vi "Dashboard Main.vi"() -> ()   [LabVIEW 2014]
uses:
  <vilib>/event_ctls.llb/eventvkey.ctl
  <vilib>/Rock Robotics/WPI/Dashboard/WPI_DashboardLogging Global.vi
  <vilib>/Rock Robotics/Network Tables/SD Write Number.vi
  <vilib>/Rock Robotics/Network Tables/SD Write Boolean.vi
  <vilib>/Rock Robotics/Network Tables/SD Read String.vi
  <vilib>/Utility/config.llb/Write Key (String).vi
  <vilib>/Utility/config.llb/Write Key (I32).vi
  <vilib>/Utility/config.llb/NI_LVConfig.lvlib
panel:
  in  "TCP":refnum<k5>
  in  "Rec Mode":enum32{"Stop", "Record", "Playback"}(radio)
  in  "Vision":u16(ring) items=["Camera Off", "USB Camera SW", "USB Camera HW", "IP Camera"]
  out "Camera IP":string
  out "Image Message":string="Timeout in Camera Communications"
  in  "Dashboard Tab":T1(tab)
  in  "CPS":dbl
  in  "Precision":bool
  out "?":string
  out "?":string
  out "?":string
  out "?":string
  out "?":string
  out "?":string
  in  "?":bool
  in  "?":bool
  in  "?":bool
  in  "Precision":dbl(slide) scale=0.0..100.0
  in  "Camera Settings":T2={"Frame Rate"=30, "Compression"=30, "Size"=1} {"Frame Rate" scale=1.0..30.0; "Size" items=["640x480", "320x240", "160x120"]}
  out "MotorChart R":cluster{"Numeric":dbl, "Numeric":dbl}(graph)
  out "MotorChart L":T3(graph)
  out "MotorSliders R":cluster{"MotorSlide1":dbl, "MotorSlide2":dbl} {"MotorSlide2" scale=-1.0..1.0 scale format="%#_2e"; "MotorSlide1" scale=-1.0..1.0 scale format="%#_2e"}
  out "MotorSliders L":T4 {"MotorSlide4 2" scale=0.0..14.0 scale format="%#_2e"; "MotorSlide2" scale=-1.0..1.0 scale format="%#_2e"; "MotorSlide1" scale=-1.0..1.0 scale format="%#_2e"}
  out "?":dbl(knob) scale=0.0..360.0
  out "JS1 Z":dbl(slide) scale=-1.0..1.0 scale format="%#_2e"
  out "JS1 Graph":cluster{"X":dbl, "Y":dbl}[](graph)
  out "JS1 Buttons":T5
  out "JS2 Z":dbl(slide) scale=-1.0..1.0 scale format="%#_2e"
  out "JS2 Graph":cluster{"X":dbl, "Y":dbl}[](graph)
  out "JS2 Buttons":T5
  out "Mode":T6(ring)=enum."Auto Disabled"
  in  "DB Camera Config":bool
  out "fps":dbl format="%#.1g"
  out "Mbps":dbl format="%#.1g"
  out "Mbps 2":bool
  in  "DB/String 9":string
  in  "DB/String 8":string
  in  "DB/String 7":string
  in  "DB/String 6":string
  in  "DB/String 5":string
  in  "DB/String 4":string
  in  "DB/String 3":string
  in  "DB/String 2":string
  in  "DB/String 1":string
  in  "DB/String 0":string
  in  "DB/Slider 0":dbl(slide) scale=0.0..5.0
  in  "DB/Slider 1":dbl(slide) scale=0.0..5.0
  in  "DB/Slider 2":dbl(slide) scale=0.0..5.0
  in  "DB/Slider 3":dbl(slide) scale=0.0..5.0
  out "DB/LED 3":bool
  out "DB/LED 2":bool
  out "DB/LED 1":bool
  out "DB/LED 0":bool
  in  "DB/Button 3":bool
  in  "DB/Button 2":bool
  in  "DB/Button 1":bool
  in  "DB/Button 0":bool caption="New Name"
  in  "Test Slider":dbl(slide) scale=0.0..100.0 scale format="%#_3g"
  in  "On/Off":bool caption="Solenoid"
  in  "Test Name":u16(ring) items=["Select the test to run...", "Example Test", "-------------------------------", "List of tests is built in robot code.", "Replace with your own automated tests."]
  in  "Test Tree":string(tree)
  in  "Motor":cluster{"Value":dbl, "Enable":bool} {"Value" scale=-1.0..1.0 scale format="%#_3g"}
  out "Progress":T7 {"Test Progress" scale=0.0..100.0}
  in  "Rev/Fwd":cluster{"Forward":bool, "Reverse":bool}
  in  "Test Ring":u16(ring) items=["Monochrome", "Color"]
  in  "Listbox":i32(listbox)
  out "Tree":string(tree)
  in  "Invert Z":bool
  in  "Invert Y":bool
  in  "Invert X":bool
  out "Camera Image":T8(plugin-control)
  out "Boolean":bool
  # "Left"
  # "Front"
  # "Right"
  # "Battery"
  # "This tab is a great place for autonomous settings and robot-specific values.\nPlace controls and indicators inside this tab and match name to\nDashboard Variables on robot. You can also delete this comment."
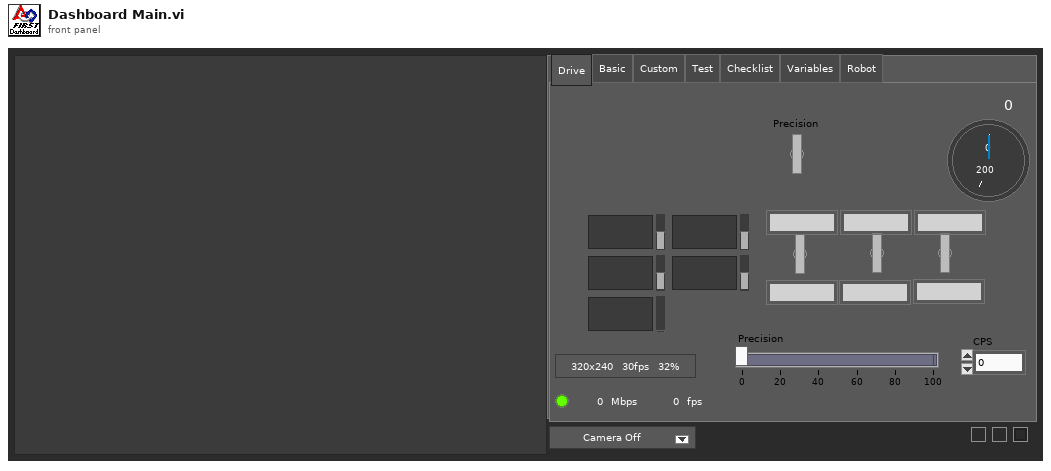
[diagram p1: front panel]
types:
  T1 = enum32{"Drive", "Basic", "Custom", "Test", "Checklist", "Variables", "Robot"}
  T2 = cluster{"Frame Rate":i32, "Compression":i32, "Size":u16}
  T3 = cluster{"Numeric":dbl, "Numeric":dbl, "Battery V":dbl}
  T4 = cluster{"MotorSlide1":dbl, "MotorSlide2":dbl, "MotorSlide4 2":dbl}
  T5 = cluster{bool, bool, bool, bool, bool, bool, bool, bool, bool, bool, bool, bool}
  T6 = enum8{"Tele-Op Disabled", "Tele-Op Enabled", "Auto Disabled", "Auto Enabled", "Test Disabled", "Test Enabled", "Disconnected", "No Code", "E-Stop"}
  T7 = cluster{"Test Progress":u8, "Test Progress Text":string}
  T8 = typedef "IMAQ Image.ctl" = refnum<image>
  T9 = enum32{"Drive", "Basic", "Custom", "Test", "Checklist", "Variables"}
  T10 = typedef "Image Type" = u32
  T11 = cluster{"Camera Image":refnum<vi>, "Dashboard Tab":refnum<vi>, "Boolean":refnum<vi>, "Vision":refnum<vi>, "Rec Mode":refnum<vi>, "Test Slider":refnum<vi>, "On/Off ":refnum<vi>, "Test Ring":refnum<vi>, "Rev/Fwd":refnum<vi>, "Test Name":refnum<vi>, "Motor":refnum<vi>, "Progress":refnum<vi>, "CheckList":refnum<vi>, "Tree":refnum<vi>, "Test Tree":refnum<vi>}
  T12 = typedef "NI_LVConfig.lvlib/Config Data RefNum.ctl" = refnum<k1>
  T13 = cluster{"Error Strings":string, "Disable Counts":cluster{u16, u16}, "Rail Faults":cluster{u16, u16, u16}, "Robot IP":string, "DB Mode":u8, "Event Info":cluster{"Name":string, "Type":u8, "Number":u16, "Replay":u8}, "Camera Addr":string}
  T14 = cluster{"Storage":cluster{"Disk Free":u64, "RAM Block":u32, "RAM free":u32}, "CPU Utilization":cluster{"CPU % ISR":sgl, "CPU % Time Crit":sgl, "CPU % Timed Str":sgl, "CPU % High":sgl, "CPU % Above":sgl, "CPU % Normal":sgl, "CPU % Low":sgl}, "CAN":cluster{"% Bus Utilization":sgl, "Bus Off Cnt":u32, "TX_FIFO Full Cnt":u32, "Receive Error Cnt":u8, "Transmit Error Cnt":u8}, "HID":cluster{"HID Outputs":u32, "Rumble Low":u16, "Rumble High":u16}[]}
  T15 = cluster{"Status bits":cluster{"Test Mode":bool, "Autonomous":bool, "Enabled":bool, "Code Start":bool, "Brownout":bool, "Reserved 2":bool, "Reserved 3":bool, "E-Stop":bool}, "Code Trace":cluster{"Disabled":bool, "TeleOp":bool, "Auto":bool, "Test":bool}, "Controller Type":enum16{"unknown", "cRIO", "roboRio"}, "Code?":enum16{"unknown", "noCode", "code"}, "Battery V":dbl}
  T16 = cluster{"Control Bits":cluster{"TestMode":bool, "Autonomous":bool, "Enabled":bool, "FMS Present":bool, bool, bool, bool, "E-Stop":bool}, "Team Station ":u8, "Countdown":sgl, "Joystick Values":cluster{"Axes":dbl[], "Buttons":bool[], "POVs":i16[]}[]}
  T17 = cluster{"Axes":dbl[], "Buttons":bool[], "POVs":i16[]}[]
  T18 = cluster{"Axes":dbl[], "Buttons":bool[], "POVs":i16[]}
  T19 = cluster{"Buttons[0]":bool, "Buttons[1]":bool, "Buttons[2]":bool, "Buttons[3]":bool, "Buttons[4]":bool, "Buttons[5]":bool, "Buttons[6]":bool, "Buttons[7]":bool, "Buttons[8]":bool, "Buttons[9]":bool, "Buttons[10]":bool, "Buttons[11]":bool}
  T20 = cluster{"Operation":enum16{"Update", "Clear"}, "Color Box":u32}[]
  T21 = typedef "eventvkey.ctl" = enum16{"ASCII", "Enter", "Return", "Shift", "Ctrl", "Alt", "Cmd", "Opt", "Caps", "NumLock", "Clear", "Break", "Up", "Down", "Left", "Right", "Insert", "Delete", "Home", "End", "PageUp", "PageDown", "Escape", "Help", "Pause", "ScrollLock", "F1", "F2", "F3", "F4", "F5", "F6", "F7", "F8", "F9", "F10", "F11", "F12", "F13", "F14", "F15", "F16", "F17", "F18", "F19", "F20", "F21", "F22", "F23", "F24", "Play", "VolumeUp", "VolumeDown", "Mute", "Two Byte Char"}
  T22 = cluster{"Image Size":bool, "Image Type":bool, "Pixel Value":bool, "ROI Information":bool, "Zoom Factor":bool}
  T23 = enum8{"Enabled", "Disabled", "Disabled and Grayed Out"}
  T24 = cluster{"Operation":enum16{"Update", "Clear"}, "Color Box":u32}
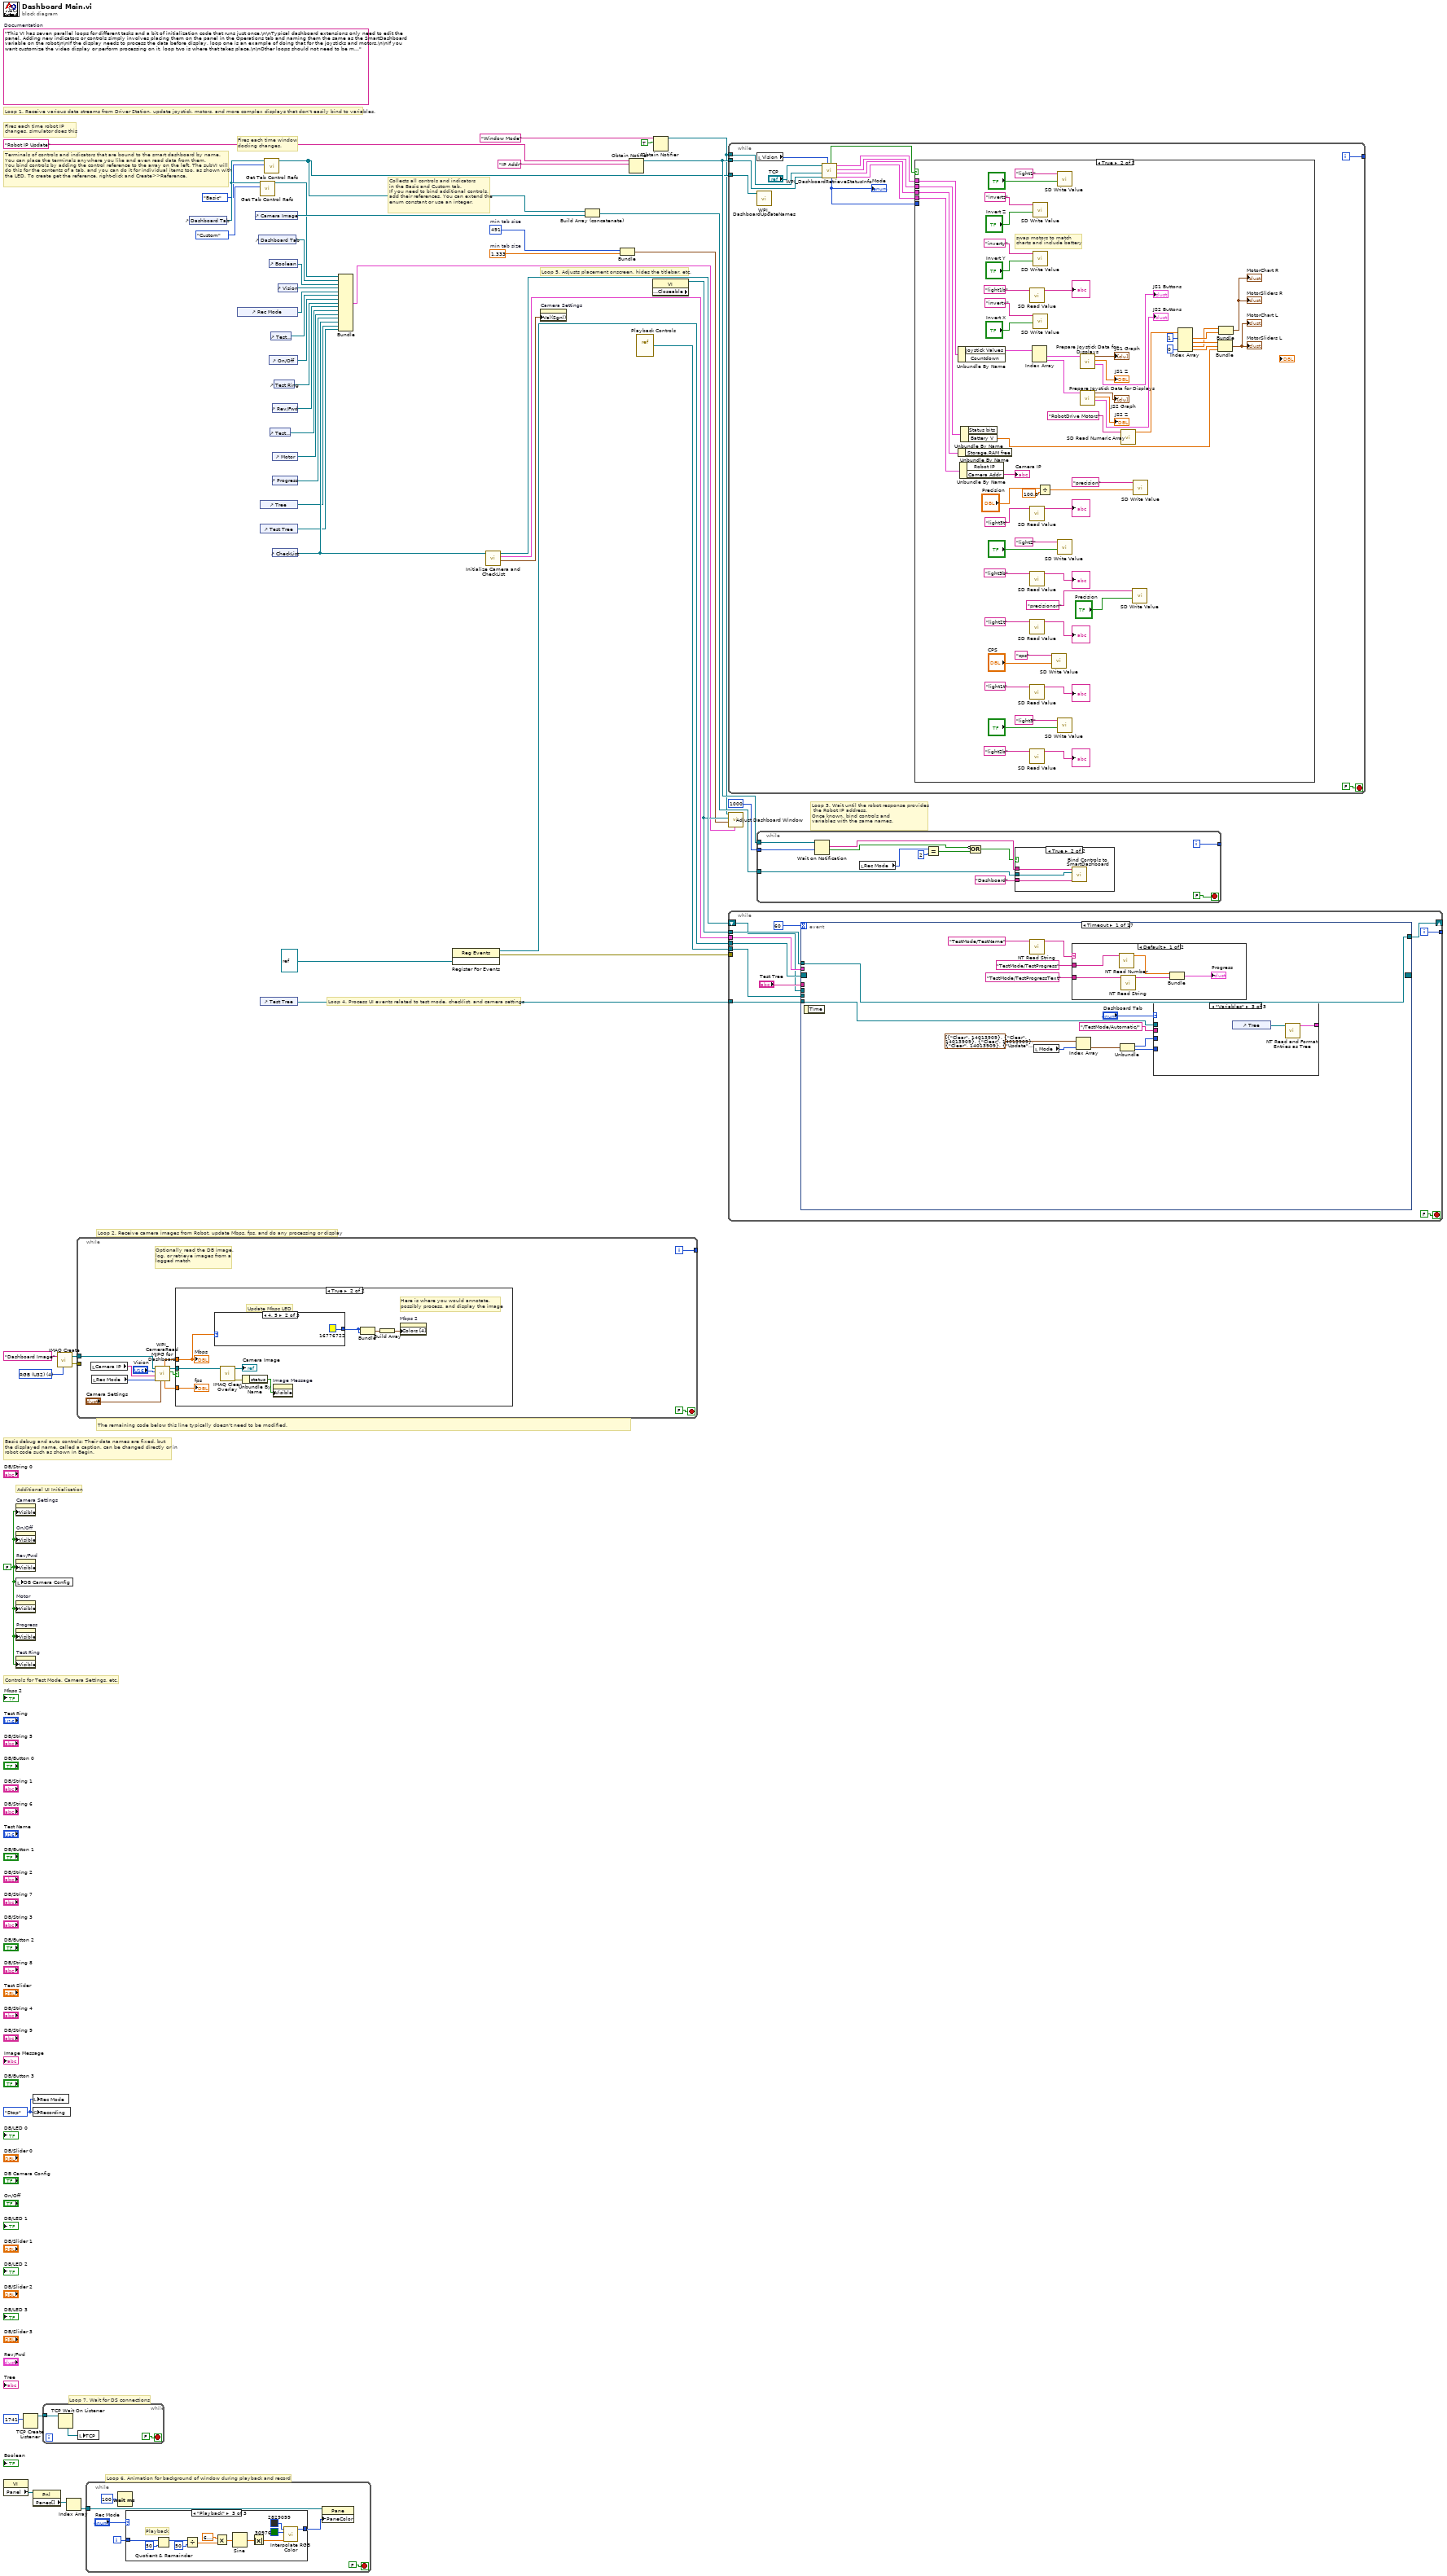
[diagram p0: block diagram]
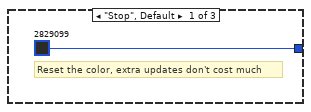
[diagram p3: hidden frame]
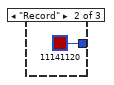
[diagram p4: hidden frame]
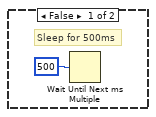
[diagram p6: hidden frame]
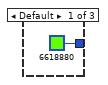
[diagram p7: hidden frame]
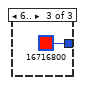
[diagram p8: hidden frame]
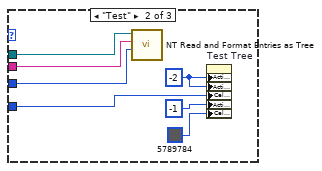
[diagram p10: hidden frame]
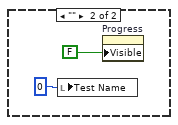
[diagram p11: hidden frame]
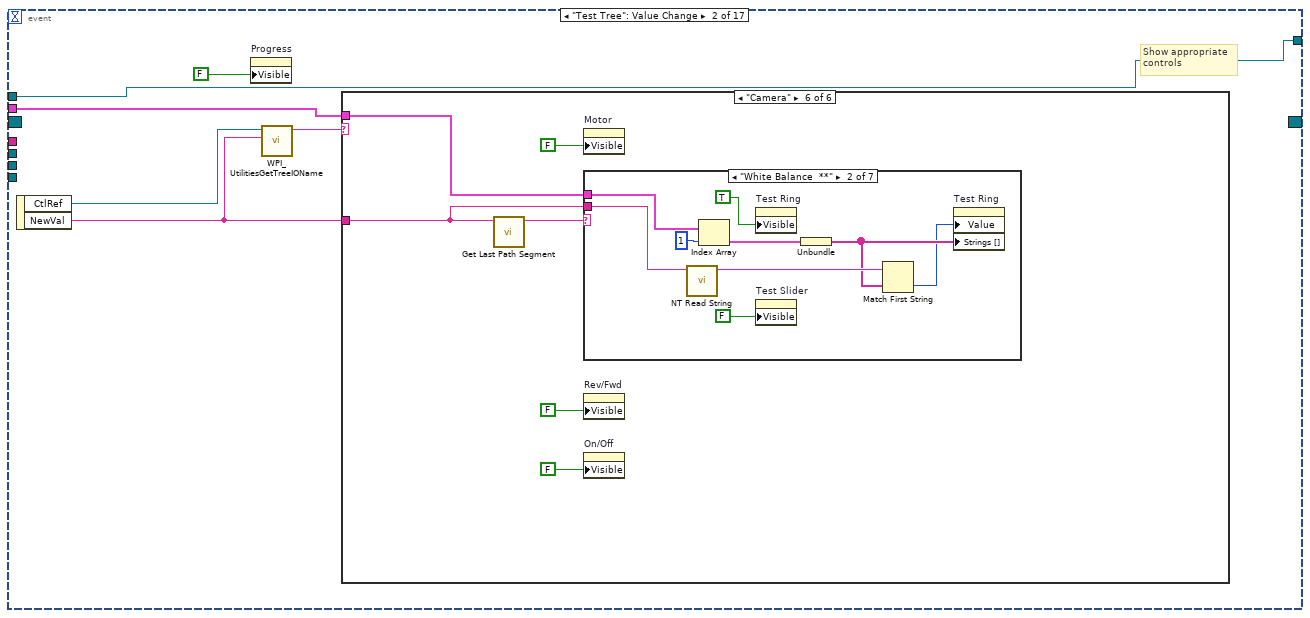
[diagram p12: hidden frame]
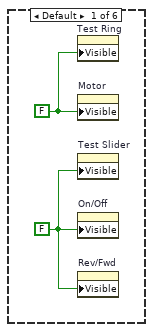
[diagram p13: hidden frame]
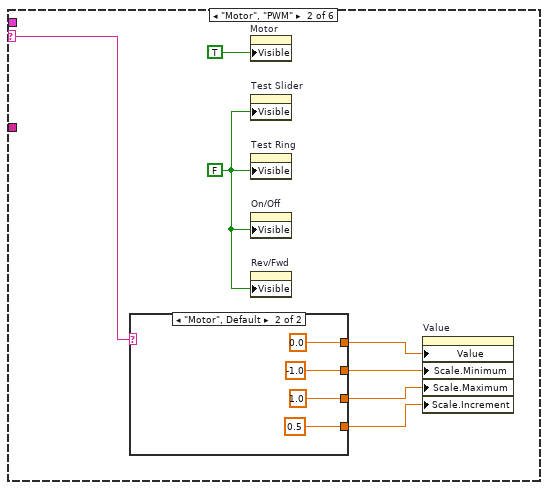
[diagram p14: hidden frame]
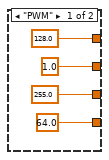
[diagram p15: hidden frame]
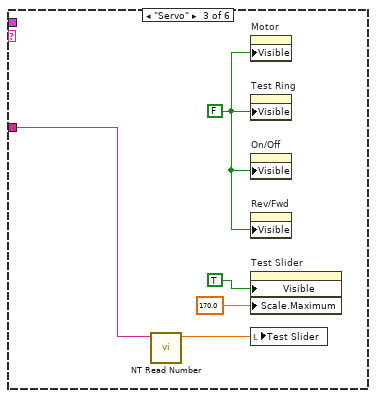
[diagram p16: hidden frame]
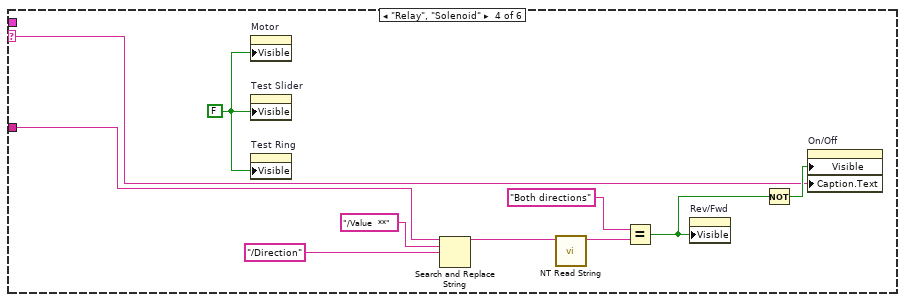
[diagram p17: hidden frame]
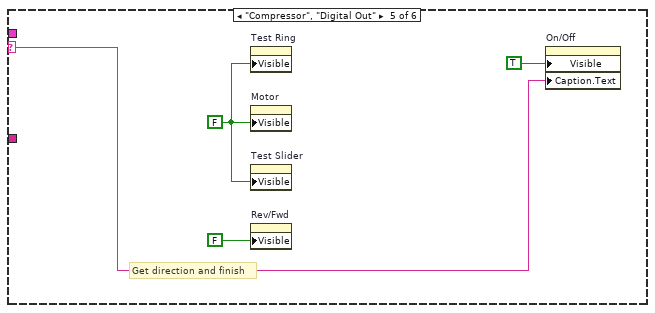
[diagram p18: hidden frame]
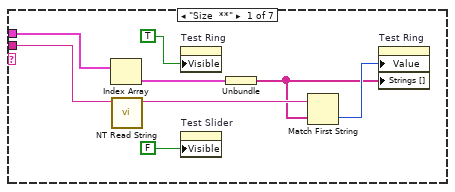
[diagram p19: hidden frame]
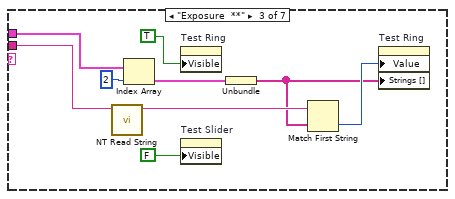
[diagram p20: hidden frame]
diagram:
  w24 = 491  # min tab size
  w23 = 1.333  # min tab size
  w32 = enum32{"Stop", "Record", "Playback"}."Stop" ("Rec Mode")
  w6 = FALSE ("Visible")
  (unwired) "This VI has seven parallel loops for different tasks and a bit of initialization code that runs just once.\n\nTypical dashboard extensions only need to edit the panel. Adding new indicators or controls simply involves placing them on the panel in the Operations tab and naming them the same as the SmartDashboard variable on the robot\n\nIf the display needs to process the data before display, loop one is an example of doing that for the joysticks and motors.\n\nIf you want customize the video display or perform processing on it, loop two is where that takes place.\n\nOther loops should not need to be modified. They are pretty standard, and document the task they perform."  # Documentation
  w52 = T10 4 items=["Grayscale (U8)", "Grayscale (I16)", "Grayscale (SGL)", "Complex (CSG)", "RGB (U32)", "HSL (U32)", "RGB (U64)"] ("Image Type")
  # "Loop 7. Wait for DS connections"
  # "Basic debug and auto controls: Their data names are fixed, but\nthe displayed name, called a caption, can be changed directly or in\nrobot code such as shown in Begin."
  # "Controls for Test Mode, Camera Settings, etc."
  # "Additional UI Initialization"
  # "Loop 6. Animation for background of window during playback and record"
  # "Fires each time robot IP\nchanges, simulator does this"
  # "Fires each time window\ndocking changes."
  # "Collects all controls and indicators\nin the Basic and Custom tab.\nIf you need to bind additional controls,\nadd their references. You can extend the\nenum constant or use an integer."
  # "The remaining code below this line typically doesn't need to be modified."
  # "Loop 4. Process UI events related to test mode, checklist, and camera settings"
  # "Terminals of controls and indicators that are bound to the smart dashboard by name.\nYou can place the terminals anywhere you like and even read data from them.\nYou bind controls by adding the control reference to the array on the left. The subVI will\ndo this for the contents of a tab, and you can do it for individual items too, as shown with\nthe LED. To create get the reference, right-click and Create>>Reference."
  # "Loop 3. Wait until the robot response provides\n the Robot IP address.\nOnce known, bind controls and\nvariables with the same names."
  # "Loop 5. Adjusts placement onscreen, hides the titlebar, etc."
  # "Loop 1. Receive various data streams from Driver Station, update joystick, motors, and more complex displays that don't easily bind to variables."
  # "Loop 2. Receive camera images from Robot, update Mbps, fps, and do any processing or display"
  n1 = property class="VI"() -> ("Panel"=w39:refnum<vi>)  [unwired: 2 in, 2 out]
  n2 = property on="Camera Settings" class="Clust (strict)"("Visible"=w6) -> ()  [unwired: 2 in, 2 out]
  n3 = property on="On/Off" class="Bool (strict)"("Visible"=w6) -> ()  [unwired: 2 in, 2 out]
  n4 = property on="Rev/Fwd" class="Clust (strict)"("Visible"=w6) -> ()  [unwired: 2 in, 2 out]
  n5 = local write "DB Camera Config"(w6) -> ()
  n6 = property on="Motor" class="Clust (strict)"("Visible"=w6) -> ()  [unwired: 2 in, 2 out]
  n7 = property on="Progress" class="Clust (strict)"("Visible"=w6) -> ()  [unwired: 2 in, 2 out]
  n8 = property on="Test Ring" class="Ring (strict)"("Visible"=w6) -> ()  [unwired: 2 in, 2 out]
  n9 = TCP Create Listener(10:u16 1741 ("timeout ms (25000)")) -> (3:w1:refnum<k5>)  [unwired: 4 in, 2 out]
  n10 = local write "Rec Mode"(w32) -> ()
  n11 = global write "WPI_DashboardLogging Global.vi" "Recording"(w32) -> ()
  n12 = property class="Pnl"(reference=w39) -> ("Panes[]"=w40:refnum<vi>[])  [unwired: 1 in, 2 out]
  n13 = while {
    tunnel: w1 -> [w54]
    stop <- FALSE stop-if-true
    n14 = TCP Wait On Listener(11:w54) -> (4:w53:refnum<k5>)  [unwired: 3 in, 4 out]
    n15 = local write "TCP"(w53) -> ()
  }
  n16 = call "IMAQ Create"("Image Name"="Dashboard Image", "Image Type"=w52) -> ("New Image"=w50:T8, "error out"=w49:errorcluster)  [unwired: 2 in, 1 out]
  n17 = Index Array(array=w40) -> (element=w38:refnum<vi>)  [unwired: 1 in]
  n18 = while {
    tunnel: w50 -> [w64]
    tunnel: w49 -> [_]
    tunnel: [w65] -> _
    i -> [w65]
    stop <- FALSE stop-if-true
    # "Optionally read the DB image,\nlog, or retrieve images from a\nlogged match"
    n19 = local read "Camera IP"() -> (w56:string)
    n20 = local read "Rec Mode"() -> (w58:enum32{"Stop", "Record", "Playback"})
    n21 = call <vilib>:"WPI_CameraRead MJPG for Dashboard.vi"("Camera Settings"="Camera Settings", "Rec Mode"=w58, "Camera IP"=w56, "Camera Mode"="Vision", "Refnum in"=w64) -> ("Active"=w62:bool, "Refnum out"=w63:T8, "FPS"=w61:dbl, "Bandwidth (Mbps)"=w60:dbl)  [unwired: 3 in]
    n22 = case shown="True" w62 {
      tunnel: w63 -> [_ w71]
      tunnel: w60 -> [_ w70]
      tunnel: w61 -> [_ w68]
      frame False {
        # "Sleep for 500ms"
        n23 = Wait Until Next ms Multiple(millisecond multiple=u32 500) -> ()  [unwired: 1 out]
      }
      frame True {
        # "Here is where you would annotate,\npossibly process, and display the image"
        # "Update Mbps LED"
        n24 = case shown="4, 5" w70 {
          tunnel: [u32 6618880 ("Color Box") u32 16776722 ("Color Box") u32 16716800 ("Color Box")] -> w72
          frame Default {
          }
          frame 4, 5 {
          }
          frame 6.. {
          }
        }
        n25 = call "IMAQ Clear Overlay"("Image"=w71) -> ("error out"=w75:errorcluster, "Image Out"=→"Camera Image":T8)  [unwired: 2 in, 7 out]
        n26 = Unbundle By Name(w75) -> ("status"=w76:bool)
        n27 = property on="Image Message" class="Str"("Visible"=w76) -> ()  [unwired: 2 in, 2 out]
        n28 = Bundle("Color Box"=w72, "Color Box"=w72) -> (w74:cluster{"Color Box":u32, "Color Box":u32})  [unwired: 1 out]
        n29 = Build Array(w74) -> (w73:cluster{"Color Box":u32, "Color Box":u32}[])
        n30 = property on="Mbps 2" class="Bool (strict)"("Colors [4]"=w73) -> ()  [unwired: 2 in, 2 out]
        "Mbps" <- w70
        "fps" <- w68
      }
    }
  }
  n31 = while {
    tunnel: w38 -> [w81]
    i -> [w84]
    stop <- FALSE stop-if-true
    n32 = Wait (ms)(milliseconds to wait=u32 100) -> ()  [unwired: 1 out]
    n33 = case shown="\"Playback\"" "Rec Mode" {
      tunnel: w84 -> [_ _ w99]
      tunnel: [u32 2829099 ("Base Color") u32 11141120 ("Target Color") w88] -> w80
      frame "Stop", Default {
        # "Reset the color, extra updates don't cost much"
      }
      frame "Record" {
      }
      frame "Playback" {
        # "Playback"
        n34 = Quotient & Remainder(x=w99, y=u32 50 ("milliseconds to wait")) -> (x-y*floor(x/y)=w95:u32)  [unwired: 1 out]
        n35 = Divide(x=w95, y=u32 50 ("milliseconds to wait")) -> (x/y=w92:dbl)
        n36 = Multiply(x=6.283185307179586, y=w92) -> (x*y=w97:dbl)
        n37 = Sine(x=w97) -> (sin(x)=w96:dbl)
        n38 = Absolute Value(x=w96) -> (abs(x)=w89:dbl)
        n39 = call "Interpolate RGB Color.vi"("Proportion"=w89, "Target Color"=u32 30976, "Base Color"=u32 2829099) -> ("Result Color"=w88:u32)  [unwired: 8 in]
      }
    }
    n40 = property class="Pane"(reference=w81, "PaneColor"=w80) -> ()  [unwired: 1 in, 2 out]
  }
  n41 = control-ref of="Dashboard Tab"() -> (w30:refnum<vi>)
  n42 = control-ref of="Rec Mode"() -> (w12:refnum<vi>)
  n43 = control-ref of="Camera Image"() -> (w27:refnum<vi>)
  n44 = control-ref of="Dashboard Tab"() -> (w26:refnum<vi>)
  n45 = control-ref of="Tree"() -> (w16:refnum<vi>)
  n46 = control-ref of="Test Tree"() -> (w15:refnum<vi>)
  n47 = control-ref of="Test Tree"() -> (w41:refnum<vi>)
  n48 = call <vilib>:"Get Tab Control Refs.vi"("Page Index"=T9."Custom" ("Dashboard Tab"), "TabControl in"=w30) -> ("ControlsOnPage"=w29:refnum<vi>[])  [unwired: 9 in]
  n49 = call <vilib>:"Get Tab Control Refs.vi"("Page Index"=T9."Basic" ("Dashboard Tab"), "TabControl in"=w30) -> ("ControlsOnPage"=w4:refnum<vi>[])  [unwired: 9 in]
  n50 = control-ref of="Boolean"() -> (w21:refnum<vi>)
  n51 = control-ref of="On/Off"() -> (w10:refnum<vi>)
  n52 = control-ref of="Test Name"() -> (w14:refnum<vi>)
  n53 = control-ref of="Test Slider"() -> (w11:refnum<vi>)
  n54 = control-ref of="Rev/Fwd"() -> (w8:refnum<vi>)
  n55 = control-ref of="Motor"() -> (w13:refnum<vi>)
  n56 = control-ref of="Progress"() -> (w7:refnum<vi>)
  n57 = control-ref of="CheckList"() -> (w17:refnum<vi>)
  n58 = control-ref of="Test Ring"() -> (w9:refnum<vi>)
  n59 = control-ref of="Vision"() -> (w25:refnum<vi>)
  n60 = Bundle("Camera Image"=w27, "Dashboard Tab"=w26, "Boolean"=w21, "Vision"=w25, "Rec Mode"=w12, "Test Slider"=w11, "On/Off"=w10, "Test Ring"=w9, "Rev/Fwd"=w8, "Test Name"=w14, "Motor"=w13, "Progress"=w7, "CheckList"=w17, "Tree"=w16, "Test Tree"=w15) -> (w18:T11)  [unwired: 1 in]
  n61 = register-events(refnum<vi> refnum) -> (reference out=w36:refnum<event-registration>, error out=w35:errorcluster)  [unwired: 2 in]
  n62 = call "Initialize Camera and CheckList.vi"("ListBox in"=w17) -> ("Cluster"=w43:cluster{"value":i32, "value":i32, "index":i32}, "Array"=w44:cluster{string[]}[], "File Refnum"=w42:T12)  [unwired: 8 in]
  n63 = property on="Camera Settings" class="Clust (strict)"("Val(Sgnl)"=w43) -> ()  [unwired: 2 in, 2 out]
  n64 = Build Array (concatenate)(w4, w29) -> (w28:refnum<vi>[])
  n65 = Bundle("min tab size"=w24, "min tab size"=w23) -> (w22:cluster{"min tab size":i32, "min tab size":dbl})  [unwired: 1 in]
  n66 = Obtain Notifier(name (unnamed)="Robot IP Update", notification data type="IP Addr" ("name (unnamed)")) -> (notifier out=w5:refnum<notifier>)  [unwired: 2 in, 2 out]
  n67 = vi-ref "Playback Controls.vi"() -> (w37:refnum<vi>)
  n68 = property class="VI" props=["Front Panel.Closeable"]() -> (reference out=w31:refnum<vi>)  [unwired: 2 in, 2 out]
  n69 = Obtain Notifier(name (unnamed)="Window Mode", notification data type=TRUE) -> (notifier out=w3:refnum<notifier>)  [unwired: 2 in, 2 out]
  n70 = while {
    tunnel: [w111] -> _
    tunnel: w5 -> [w105]
    tunnel: w4 -> [w104]
    tunnel: w3 -> [w100]
    i -> [w111]
    stop <- FALSE stop-if-true
    n71 = local read "Vision"() -> (w102:u16)
    n72 = call <vilib>:"WPI_DashboardUpdateNames.vi"("Controls on Tab"=w104) -> ()  [unwired: 11 in]
    n73 = call <vilib>:"WPI_DashboardRetrieveStatusInfo.vi"("Vision"=w102, "Binding Refnum"=w105, "Window Mode Notifier"=w100, "TCP Cnx"="TCP") -> ("Power and Errors"=w106:T13, "Robot Metrics"=w109:T14, "Status Info"=w110:T15, "Control Info"=w107:T16, "Robot Mode"=w103:T6, "Process?"=w108:bool)  [unwired: 2 in]
    "Mode" <- w103
    n74 = case shown="True" w108 {
      tunnel: w110 -> [_ w169]
      tunnel: w109 -> [_ w168]
      tunnel: w107 -> [_ w167]
      tunnel: w106 -> [_ w166]
      tunnel: w103 -> [_ _]
      frame False {
      }
      frame True {
        # "swap motors to match\ncharts and include battery"
        n75 = Unbundle By Name(w167) -> ("Joystick Values"=w154:T17)  [unwired: 1 out]
        n76 = Unbundle By Name(w168) -> ()  [unwired: 1 out]
        n77 = Unbundle By Name(w166) -> ("Camera Addr"=→"Camera IP":string)  [unwired: 1 out]
        n78 = Unbundle By Name(w169) -> ("Battery V"=w155:dbl)  [unwired: 1 out]
        n79 = call-poly <vilib>:"SD Read Value.vi"("Name"="light1b") -> ("String"=→"?":string)  [unwired: 8 in, 2 out]
        n80 = call-poly <vilib>:"SD Read Value.vi"("Name"="light3t") -> ("String"=→"?":string)  [unwired: 8 in, 2 out]
        n81 = call-poly <vilib>:"SD Read Value.vi"("Name"="light3b") -> ("String"=→"?":string)  [unwired: 8 in, 2 out]
        n82 = call-poly <vilib>:"SD Read Value.vi"("Name"="light2t") -> ("String"=→"?":string)  [unwired: 8 in, 2 out]
        n83 = call-poly <vilib>:"SD Read Value.vi"("Name"="light1t") -> ("String"=→"?":string)  [unwired: 8 in, 2 out]
        n84 = call-poly <vilib>:"SD Read Value.vi"("Name"="light2b") -> ("String"=→"?":string)  [unwired: 8 in, 2 out]
        n85 = Index Array(array=w154) -> (element #1=w153:T18, element #2=w148:T18)  [unwired: 2 in]
        n86 = call-poly <vilib>:"SD Write Value.vi"("Boolean"="Invert Z", "Name"="invertz") -> ()  [unwired: 8 in, 2 out]
        n87 = call-poly <vilib>:"SD Write Value.vi"("Boolean"="Invert Y", "Name"="inverty") -> ()  [unwired: 8 in, 2 out]
        n88 = call-poly <vilib>:"SD Write Value.vi"("Boolean"="Invert X", "Name"="invertx") -> ()  [unwired: 8 in, 2 out]
        n89 = Divide(x="Precision", y=100.0) -> (x/y=w143:dbl)
        n90 = call-poly <vilib>:"SD Write Value.vi"("Numeric"="CPS", "Name"="cps") -> ()  [unwired: 8 in, 2 out]
        n91 = call-poly <vilib>:"SD Write Value.vi"("Boolean"="?", "Name"="light1") -> ()  [unwired: 8 in, 2 out]
        n92 = call-poly <vilib>:"SD Write Value.vi"("Boolean"="?", "Name"="light2") -> ()  [unwired: 8 in, 2 out]
        n93 = call-poly <vilib>:"SD Write Value.vi"("Boolean"="?", "Name"="light3") -> ()  [unwired: 8 in, 2 out]
        n94 = call "Prepare Joystick Data for Displays.vi"("Joystick Values"=w153) -> ("Buttons"=→"JS1 Buttons":T19, "Z Axis"=→"JS1 Z":dbl, "Cartesian Data"=→"JS1 Graph":cluster{"X axis":dbl, "X axis":dbl}[])  [unwired: 8 in]
        n95 = call "Prepare Joystick Data for Displays.vi"("Joystick Values"=w148) -> ("Buttons"=→"JS2 Buttons":T19, "Z Axis"=→"JS2 Z":dbl, "Cartesian Data"=→"JS2 Graph":cluster{"X axis":dbl, "X axis":dbl}[])  [unwired: 8 in]
        n96 = call <vilib>:"SD Read Numeric Array.vi"("Name"="RobotDrive Motors") -> ("Numeric Array"=w157:dbl[])  [unwired: 8 in, 2 out]
        n97 = call-poly <vilib>:"SD Write Value.vi"("Boolean"="Precision", "Name"="precisionon") -> ()  [unwired: 8 in, 2 out]
        n98 = call-poly <vilib>:"SD Write Value.vi"("Numeric"=w143, "Name"="precision") -> ()  [unwired: 8 in, 2 out]
        n99 = Index Array(array=w157, index #1=1, index #4=0) -> (element #1=w161:dbl, element #2=w162:dbl, element #3=w160:dbl, element #4=w165:dbl)  [unwired: 2 in]
        n100 = Bundle("Numeric"=w162, "Numeric"=w165, "Battery V"=w155) -> (→"MotorChart L" →"MotorSliders L":T3)  [unwired: 1 in]
        n101 = Bundle("Numeric"=w160, "Numeric"=w161) -> (→"MotorChart R" →"MotorSliders R":cluster{"Numeric":dbl, "Numeric":dbl})  [unwired: 1 in]
      }
    }
  }
  n102 = call "Adjust Dashboard Window.vi"("Sizing Refnums"=w18, "Size Constraints"=w22, "VI"=w31, "Notifier in"=w3) -> ()  [unwired: 8 in]
  n103 = while {
    tunnel: w44 -> [w177]
    shift-right: [w176] -> _
    shift-left: w42 -> [w175]
    tunnel: [w174] -> _
    tunnel: w41 -> [w173]
    tunnel: w37 -> [w172]
    tunnel: w36 -> [w171]
    tunnel: w35 -> [_]
    tunnel: w31 -> [w170]
    i -> [w174]
    stop <- FALSE stop-if-true
    n104 = event shown="[0] Timeout" {
      selector: w171 -> [_ _ _ _ _ _ _ _ _ _ _ _ _ _ _ _ _]
      dyn-events: [_ _ _ _ _ _ _ _ _ _ _ _ _ w415 _ _ _] -> _
      timeout: u32 60 ("milliseconds to wait") -> [_ _ _ _ _ _ _ _ _ _ _ _ _ _ _ _ _]
      tunnel: w173 -> [w189 _ _ _ _ _ _ _ _ _ _ _ _ _ _ _ _]
      tunnel: "Test Tree" -> [_ _ _ _ _ _ _ _ w384 w392 w394 w398 w406 _ _ _ _]
      tunnel: w177 -> [_ w211 _ _ _ _ w348 w378 _ _ _ _ _ _ _ _ _]
      tunnel: [w185 w210 w309 w314 w322 w334 w347 w371 w383 w390 w393 w397 w405 w417 w431 w432 w442] -> w176
      tunnel: w175 -> [w185 w210 w309 w314 w322 w334 w346 w371 w383 w390 w393 w397 w405 w417 w431 w432 w442]
      tunnel: w172 -> [_ _ _ _ _ _ _ _ _ _ _ _ _ w418 _ w435 _]
      tunnel: w170 -> [_ _ _ _ _ _ _ _ _ _ _ _ _ w413 _ _ _]
      event Timeout {
        n105 = event-data() -> ()  [unwired: 1 in, 1 out]
        n106 = call <vilib>:"NT Read String.vi"("Name"="TestMode/TestName") -> ("String"=w192:string)  [unwired: 9 in, 1 out]
        n107 = local read "Mode"() -> (w188:T6)
        n108 = case shown="Default" w192 {
          tunnel: "TestMode/TestProgress" ("Name") -> [w204 _]
          tunnel: "TestMode/TestProgressText" ("Name") -> [w203 _]
          frame Default {
            n109 = call <vilib>:"NT Read Number.vi"("Name"=w204) -> ("Numeric"=w205:dbl)  [unwired: 9 in, 1 out]
            n110 = call <vilib>:"NT Read String.vi"("Name"=w203) -> ("String"=w206:string)  [unwired: 9 in, 1 out]
            n111 = Bundle("Numeric"=w205, "String"=w206) -> (→"Progress":cluster{"Numeric":dbl, "String":string})  [unwired: 1 in]
          }
          frame "" {
            n112 = local write "Test Name"(u16 0) -> ()
            n113 = property on="Progress" class="Clust (strict)"("Visible"=FALSE) -> ()  [unwired: 2 in, 2 out]
          }
        }
        n114 = Index Array(array=T20 [{"Operation"=enum."Clear", "Color Box"=14013909}, {"Operation"=enum."Clear", "Color Box"=14013909}, {"Operation"=enum."Clear", "Color Box"=14013909}, {"Operation"=enum."Clear", "Color Box"=14013909}, {"Operation"=enum."Update", "Color Box"=14013909}, {"Operation"=enum."Update", "Color Box"=16777215}, {"Operation"=enum."Clear", "Color Box"=14013909}, {"Operation"=enum."Clear", "Color Box"=14013909}, {"Operation"=enum."Clear", "Color Box"=14013909}], index=w188) -> (element=w183:T24)
        n115 = Unbundle(w183) -> ("Operation"=w182:enum16{"Update", "Clear"}, "Color Box"=w181:u32)
        n116 = case shown="\"Variables\"" "Dashboard Tab" {
          tunnel: w189 -> [_ w200 _]
          tunnel: "/TestMode/Automatic/" ("Name Pattern") -> [_ w199 _]
          tunnel: w182 -> [_ w198 _]
          tunnel: [_ _ w202] -> _
          tunnel: w181 -> [_ w194 _]
          frame "Custom", Default {
          }
          frame "Test" {
            w197 = -2 ("Active Item:Row Number")
            n117 = call <vilib>:"NT Read and Format Entries as Tree.vi"("Operation"=w198, "Name Pattern"=w199, "Tree Refnum"=w200) -> ()  [unwired: 7 in, 2 out]
            n118 = property on="Test Tree" class="Tree (strict)"("Active Item Row Number"=w197, "ActiveColNum"=w197, "CellBG"=w194, "Active Item Row Number"=-1 ("Active Item:Row Number"), "CellBG"=u32 5789784 ("Color Box")) -> ()  [unwired: 2 in, 2 out]
          }
          frame "Variables" {
            n119 = control-ref of="Tree"() -> (w201:refnum<vi>)
            n120 = call <vilib>:"NT Read and Format Entries as Tree.vi"("Tree Refnum"=w201) -> ("Formatted Strings"=w202:cluster{"Name":string, "Value":string}[])  [unwired: 9 in, 1 out]
          }
        }
      }
      event "Test Tree": Value Change {
        # "Show appropriate\ncontrols"
        n121 = event-data() -> ("CtlRef"=w214:refnum<vi>, "NewVal"=w212:string)  [unwired: 1 in]
        n122 = property on="Progress" class="Clust (strict)"("Visible"=FALSE) -> ()  [unwired: 2 in, 2 out]
        n123 = call <vilib>:"WPI_UtilitiesGetTreeIOName.vi"("NewVal"=w212, "TreeControl in"=w214) -> ("I/O Name"=w215:string)  [unwired: 9 in]
        n124 = case shown="\"Camera\"" w215 {
          selector: w215 -> [_ w222 _ w240 w249 _]
          tunnel: w212 -> [_ _ w237 w239 _ w256]
          tunnel: w211 -> [_ _ _ _ _ w255]
          frame Default {
            w217 = FALSE ("Visible")
            w216 = FALSE ("Visible")
            n125 = property on="Test Ring" class="Ring (strict)"("Visible"=w216) -> ()  [unwired: 2 in, 2 out]
            n126 = property on="Motor" class="Clust (strict)"("Visible"=w216) -> ()  [unwired: 2 in, 2 out]
            n127 = property on="Test Slider" class="Slide (strict)"("Visible"=w217) -> ()  [unwired: 2 in, 2 out]
            n128 = property on="On/Off" class="Bool (strict)"("Visible"=w217) -> ()  [unwired: 2 in, 2 out]
            n129 = property on="Rev/Fwd" class="Clust (strict)"("Visible"=w217) -> ()  [unwired: 2 in, 2 out]
          }
          frame "Motor", "PWM" {
            w223 = FALSE ("Visible")
            n130 = case shown="\"Motor\", Default" w222 {
              tunnel: [1.0 ("Value") -1.0 ("Value")] -> w221
              tunnel: [255.0 ("Value") 1.0 ("Value")] -> w220
              tunnel: [128.0 ("Value") 0.0 ("Value")] -> w219
              tunnel: [64.0 ("Value") 0.5 ("Value")] -> w218
              frame "PWM" {
              }
              frame "Motor", Default {
              }
            }
            n131 = property on="Motor" class="Clust (strict)"("Visible"=TRUE) -> ()  [unwired: 2 in, 2 out]
            n132 = property on="Test Slider" class="Slide (strict)"("Visible"=w223) -> ()  [unwired: 2 in, 2 out]
            n133 = property on="Test Ring" class="Ring (strict)"("Visible"=w223) -> ()  [unwired: 2 in, 2 out]
            n134 = property on="On/Off" class="Bool (strict)"("Visible"=w223) -> ()  [unwired: 2 in, 2 out]
            n135 = property on="Rev/Fwd" class="Clust (strict)"("Visible"=w223) -> ()  [unwired: 2 in, 2 out]
            n136 = property on="Value" class="Slide (strict)"("Value"=w219, "Scale.Minimum"=w221, "Scale.Maximum"=w220, "Scale.Increment"=w218) -> ()  [unwired: 2 in, 2 out]
          }
          frame "Servo" {
            w235 = FALSE ("Visible")
            n137 = call <vilib>:"NT Read Number.vi"("Name"=w237) -> ("Numeric"=w236:dbl)  [unwired: 9 in, 1 out]
            n138 = property on="Motor" class="Clust (strict)"("Visible"=w235) -> ()  [unwired: 2 in, 2 out]
            n139 = property on="Test Ring" class="Ring (strict)"("Visible"=w235) -> ()  [unwired: 2 in, 2 out]
            n140 = property on="On/Off" class="Bool (strict)"("Visible"=w235) -> ()  [unwired: 2 in, 2 out]
            n141 = property on="Rev/Fwd" class="Clust (strict)"("Visible"=w235) -> ()  [unwired: 2 in, 2 out]
            n142 = property on="Test Slider" class="Slide (strict)"("Visible"=TRUE, "Scale.Maximum"=170.0 ("Scale.Range:Maximum")) -> ()  [unwired: 2 in, 2 out]
            n143 = local write "Test Slider"(w236) -> ()
          }
          frame "Relay", "Solenoid" {
            w238 = FALSE ("Visible")
            n144 = property on="Motor" class="Clust (strict)"("Visible"=w238) -> ()  [unwired: 2 in, 2 out]
            n145 = property on="Test Slider" class="Slide (strict)"("Visible"=w238) -> ()  [unwired: 2 in, 2 out]
            n146 = property on="Test Ring" class="Ring (strict)"("Visible"=w238) -> ()  [unwired: 2 in, 2 out]
            n147 = Search and Replace String(input string=w239, search string="/Value  **", replace string="/Direction") -> (result string=w245:string)  [unwired: 5 in, 3 out]
            n148 = call <vilib>:"NT Read String.vi"("Name"=w245) -> ("String"=w243:string)  [unwired: 9 in, 1 out]
            n149 = Equal?(x="Both directions", y=w243) -> (x = y?=w241:bool)
            n150 = property on="Rev/Fwd" class="Clust (strict)"("Visible"=w241) -> ()  [unwired: 2 in, 2 out]
            n151 = Not(x=w241) -> (.not. x?=w242:bool)
            n152 = property on="On/Off" class="Bool (strict)"("Visible"=w242, "Caption.Text"=w240) -> ()  [unwired: 2 in, 2 out]
          }
          frame "Compressor", "Digital Out" {
            w248 = FALSE ("Visible")
            # "Get direction and finish"
            n153 = property on="Test Ring" class="Ring (strict)"("Visible"=w248) -> ()  [unwired: 2 in, 2 out]
            n154 = property on="Motor" class="Clust (strict)"("Visible"=w248) -> ()  [unwired: 2 in, 2 out]
            n155 = property on="Test Slider" class="Slide (strict)"("Visible"=w248) -> ()  [unwired: 2 in, 2 out]
            n156 = property on="Rev/Fwd" class="Clust (strict)"("Visible"=FALSE) -> ()  [unwired: 2 in, 2 out]
            n157 = property on="On/Off" class="Bool (strict)"("Visible"=TRUE, "Caption.Text"=w249) -> ()  [unwired: 2 in, 2 out]
          }
          frame "Camera" {
            n158 = call <vilib>:"Get Last Path Segment.vi"("String in"=w256) -> ("String out"=w257:string)  [unwired: 10 in]
            n159 = property on="Motor" class="Clust (strict)"("Visible"=FALSE) -> ()  [unwired: 2 in, 2 out]
            n160 = case shown="\"White Balance  **\"" w257 {
              tunnel: w256 -> [w263 w272 w281 w290 w299 _ w305]
              tunnel: w255 -> [w261 w269 w278 w287 w296 _ _]
              frame "Size  **" {
                n161 = Index Array(array=w261) -> (element=w260:cluster{string[]})  [unwired: 1 in]
                n162 = call <vilib>:"NT Read String.vi"("Name"=w263) -> ("String"=w262:string)  [unwired: 9 in, 1 out]
                n163 = property on="Test Ring" class="Ring (strict)"("Visible"=TRUE) -> ()  [unwired: 2 in, 2 out]
                n164 = property on="Test Slider" class="Slide (strict)"("Visible"=FALSE) -> ()  [unwired: 2 in, 2 out]
                n165 = Unbundle(w260) -> (w258:string[])
                n166 = Match First String(2:w258, 3:w262) -> (0:w259:i32)  [unwired: 1 out]
                n167 = property on="Test Ring" class="Ring (strict)"("Value"=w259, "Strings []"=w258) -> ()  [unwired: 2 in, 2 out]
              }
              frame "White Balance  **" {
                n168 = call <vilib>:"NT Read String.vi"("Name"=w272) -> ("String"=w271:string)  [unwired: 9 in, 1 out]
                n169 = Index Array(array=w269, index=1) -> (element=w270:cluster{string[]})
                n170 = property on="Test Ring" class="Ring (strict)"("Visible"=TRUE) -> ()  [unwired: 2 in, 2 out]
                n171 = property on="Test Slider" class="Slide (strict)"("Visible"=FALSE) -> ()  [unwired: 2 in, 2 out]
                n172 = Unbundle(w270) -> (w267:string[])
                n173 = Match First String(2:w267, 3:w271) -> (0:w266:i32)  [unwired: 1 out]
                n174 = property on="Test Ring" class="Ring (strict)"("Value"=w266, "Strings []"=w267) -> ()  [unwired: 2 in, 2 out]
              }
              frame "Exposure  **" {
                n175 = call <vilib>:"NT Read String.vi"("Name"=w281) -> ("String"=w280:string)  [unwired: 9 in, 1 out]
                n176 = Index Array(array=w278, index=2) -> (element=w279:cluster{string[]})
                n177 = property on="Test Ring" class="Ring (strict)"("Visible"=TRUE) -> ()  [unwired: 2 in, 2 out]
                n178 = property on="Test Slider" class="Slide (strict)"("Visible"=FALSE) -> ()  [unwired: 2 in, 2 out]
                n179 = Unbundle(w279) -> (w275:string[])
                n180 = Match First String(2:w275, 3:w280) -> (0:w276:i32)  [unwired: 1 out]
                n181 = property on="Test Ring" class="Ring (strict)"("Value"=w276, "Strings []"=w275) -> ()  [unwired: 2 in, 2 out]
              }
              frame "Exposure Priority  **" {
                n182 = call <vilib>:"NT Read String.vi"("Name"=w290) -> ("String"=w289:string)  [unwired: 9 in, 1 out]
                n183 = Index Array(array=w287, index=3) -> (element=w288:cluster{string[]})
                n184 = property on="Test Ring" class="Ring (strict)"("Visible"=TRUE) -> ()  [unwired: 2 in, 2 out]
                n185 = property on="Test Slider" class="Slide (strict)"("Visible"=FALSE) -> ()  [unwired: 2 in, 2 out]
                n186 = Unbundle(w288) -> (w284:string[])
                n187 = Match First String(2:w284, 3:w289) -> (0:w285:i32)  [unwired: 1 out]
                n188 = property on="Test Ring" class="Ring (strict)"("Value"=w285, "Strings []"=w284) -> ()  [unwired: 2 in, 2 out]
              }
              frame "Color Enable  **" {
                n189 = call <vilib>:"NT Read String.vi"("Name"=w299) -> ("String"=w298:string)  [unwired: 9 in, 1 out]
                n190 = Index Array(array=w296, index=4) -> (element=w297:cluster{string[]})
                n191 = property on="Test Ring" class="Ring (strict)"("Visible"=TRUE) -> ()  [unwired: 2 in, 2 out]
                n192 = property on="Test Slider" class="Slide (strict)"("Visible"=FALSE) -> ()  [unwired: 2 in, 2 out]
                n193 = Unbundle(w297) -> (w293:string[])
                n194 = Match First String(2:w293, 3:w298) -> (0:w294:i32)  [unwired: 1 out]
                n195 = property on="Test Ring" class="Ring (strict)"("Value"=w294, "Strings []"=w293) -> ()  [unwired: 2 in, 2 out]
              }
              frame Default {
                n196 = property on="Test Slider" class="Slide (strict)"("Visible"=FALSE) -> ()  [unwired: 2 in, 2 out]
                n197 = property on="Test Ring" class="Ring (strict)"("Visible"=FALSE) -> ()  [unwired: 2 in, 2 out]
              }
              frame "Brightness  **", "Color Level  **", "Compression  **", "FPS  **", "Sharpness  **" {
                n198 = call <vilib>:"NT Read Number.vi"("Name"=w305) -> ("Numeric"=w304:dbl)  [unwired: 9 in, 1 out]
                n199 = property on="Test Ring" class="Ring (strict)"("Visible"=FALSE) -> ()  [unwired: 2 in, 2 out]
                n200 = property on="Test Slider" class="Slide (strict)"("Visible"=TRUE, "Scale.Maximum"=100.0 ("Scale.Range:Maximum")) -> ()  [unwired: 2 in, 2 out]
                n201 = local write "Test Slider"(w304) -> ()
              }
            }
            n202 = property on="Rev/Fwd" class="Clust (strict)"("Visible"=FALSE) -> ()  [unwired: 2 in, 2 out]
            n203 = property on="On/Off" class="Bool (strict)"("Visible"=FALSE) -> ()  [unwired: 2 in, 2 out]
          }
        }
      }
      event "Test Name": Mouse Enter {
        # "Populate the ring with the list of tests"
        n204 = event-data() -> ()  [unwired: 1 in, 1 out]
        n205 = call <vilib>:"NT Read String Array.vi"("Name"="TestMode/TestList") -> ("String Array"=w313:string[])  [unwired: 9 in, 1 out]
        n206 = Build Array (concatenate)("Select the test to run...", w313) -> (w312:string[])
        n207 = property on="Test Name" class="Ring (strict)"("Strings []"=w312) -> ()  [unwired: 2 in, 2 out]
      }
      event "Test Name": Value Change {
        w315 = FALSE ("Visible")
        # "Tell the robot the test name to run"
        n208 = event-data() -> ("NewVal"=w319:u16)  [unwired: 1 in]
        n209 = property on="Test Name" class="Ring (strict)"() -> ("Strings []"=w320:string[])  [unwired: 2 in, 2 out]
        n210 = property on="Progress" class="Clust (strict)"("Visible"=TRUE) -> ()  [unwired: 2 in, 2 out]
        n211 = property on="Test Ring" class="Ring (strict)"("Visible"=w315) -> ()  [unwired: 2 in, 2 out]
        n212 = property on="Motor" class="Clust (strict)"("Visible"=w315) -> ()  [unwired: 2 in, 2 out]
        n213 = property on="Test Slider" class="Slide (strict)"("Visible"=w315) -> ()  [unwired: 2 in, 2 out]
        n214 = property on="On/Off" class="Bool (strict)"("Visible"=w315) -> ()  [unwired: 2 in, 2 out]
        n215 = property on="Rev/Fwd" class="Clust (strict)"("Visible"=w315) -> ()  [unwired: 2 in, 2 out]
        n216 = local write "Progress"(T7 {"Test Progress"=0, "Test Progress Text"=""} ("Progress")) -> ()
        n217 = Index Array(array=w320, index=w319) -> (element=w318:string)
        n218 = call <vilib>:"NT Write String.vi"("String"=w318, "Name"="TestMode/TestName") -> ()  [unwired: 9 in, 1 out]
      }
      event "Listbox": Double Click {
        # "Shift clears all"
        # "Update symbols on the listbox"
        n219 = event-data() -> ("PlatMods.Shift"=w323:bool, "Row"=w325:i32)  [unwired: 1 in]
        n220 = case shown="True" w323 {
          tunnel: w325 -> [w329 _]
          tunnel: 1 -> [w328 _]
          frame False {
            n221 = property on="Listbox" class="LstBox (strict)"() -> ("Item Symbols"=w327:i32[])  [unwired: 2 in, 2 out]
            n222 = Replace Array Subset(array=w327, new element=w328, index=w329) -> (w326:i32[])
            n223 = property on="Listbox" class="LstBox (strict)"("Item Symbols"=w326) -> ()  [unwired: 2 in, 2 out]
          }
          frame True {
            w330 = 0 ("Top Row")
            n224 = property on="Listbox" class="LstBox (strict)"() -> ("Number of Rows"=w332:u32)  [unwired: 2 in, 2 out]
            n225 = Initialize Array(0, w332) -> (w331:i32[])
            n226 = property on="Listbox" class="LstBox (strict)"("Top Row"=w330, "Value"=w330, "Item Symbols"=w331) -> ()  [unwired: 2 in, 2 out]
          }
        }
      }
      event "Listbox": Key Down {
        # "Update symbols on the listbox\nLeft and right keys check and uncheck"
        n227 = event-data() -> ("VKey"=w336:T21)  [unwired: 1 in]
        n228 = case shown="\"Left\", \"Right\"" w336 {
          selector: w336 -> [w341 _]
          tunnel: eventvkey."Left" ("VKey") -> [w339 _]
          frame "Left", "Right" {
            n229 = Equal?(x=w339, y=w341) -> (x = y?=w340:bool)
            n230 = Select(t=0, s=w340, f=1) -> (s? t:f=w342:i32)
            n231 = property on="Listbox" class="LstBox (strict)"() -> ("Item Symbols"=w345:i32[])  [unwired: 2 in, 2 out]
            n232 = Replace Array Subset(array=w345, new element=w342, index="Listbox") -> (w344:i32[])
            n233 = property on="Listbox" class="LstBox (strict)"("Item Symbols"=w344) -> ()  [unwired: 2 in, 2 out]
          }
          frame Default {
          }
        }
      }
      event "DB Camera Config": Value Change {
        # "Show or hide the cluster of controls, store in ini file"
        n234 = event-data() -> ("NewVal"=w349:bool)  [unwired: 1 in]
        n235 = case shown="False" w349 {
          tunnel: w348 -> [w358 _]
          tunnel: [w351 w369] -> w347
          tunnel: w346 -> [w350 w369]
          frame False {
            w365 = "Camera"
            w368 = FALSE ("Visible")
            n236 = property on="Camera Settings" class="Clust (strict)"("Visible"=w368) -> ()  [unwired: 2 in, 2 out]
            n237 = local write "DB Camera Config"(w368) -> ()
            n238 = local read "Camera Settings"() -> (w357:T2)
            n239 = Index Array(array=w358) -> (element=w361:cluster{string[]})  [unwired: 1 in]
            n240 = Unbundle(w361) -> (w360:string[])
            n241 = Unbundle(w357) -> ("Frame Rate"=w356:i32, "Compression"=w355:i32, "Size"=w359:u16)
            n242 = Index Array(array=w360, index=w359) -> (element=w354:string)
            n243 = call-poly <vilib>:"Write Key.vi"("section"=w365, "value"=w354, "key"="Size", "refnum"=w350) -> ("refnum out"=w367:T12)  [unwired: 2 in, 5 out]
            n244 = call-poly <vilib>:"Write Key.vi"("section"=w365, "value"=w356, "key"="FrameRate", "refnum"=w367) -> ("refnum out"=w366:T12)  [unwired: 1 in, 6 out]
            n245 = call-poly <vilib>:"Write Key.vi"("section"=w365, "value"=w355, "key"="Compression", "refnum"=w366) -> ("refnum out"=w352:T12)  [unwired: 1 in, 6 out]
            n246 = call <vilib>:"Close Config Data.vi"("refnum"=w352) -> ("file path"=w353:path)  [unwired: 2 in, 8 out]
            n247 = call <vilib>:"Open Config Data.vi"("configuration file path"=w353) -> ("refnum"=w351:T12)  [unwired: 8 in, 2 out]
          }
          frame True {
            n248 = property on="Camera Settings" class="Clust (strict)"("Visible"=TRUE) -> ()  [unwired: 2 in, 2 out]
          }
        }
      }
      event "Camera Settings": Value Change {
        # "Update summary string when any elements of DB camera change"
        n249 = event-data() -> ("NewVal"=w382:T2)  [unwired: 1 in]
        n250 = Index Array(array=w378) -> (element=w377:cluster{string[]})  [unwired: 1 in]
        n251 = Unbundle(w382) -> ("Frame Rate"=w373:i32, "Compression"=w372:i32, "Size"=w375:u16)
        n252 = Unbundle(w377) -> (w376:string[])
        n253 = Index Array(array=w376, index=w375) -> (element=w374:string)
        n254 = Format Into String(format string="%s   %dfps   %d%%", w374, w373, w372) -> (resulting string=w379:string)  [unwired: 2 in, 1 out]
        n255 = Build Array(w379) -> (w380:string[])
        n256 = property on="DB Camera Config" class="Bool (strict)"("Strings [4]"=w380) -> ()  [unwired: 2 in, 2 out]
      }
      event "Motor.Enable": Value Change {
        # "When the test mode otor enable helper is set, update that\ntree row item's value"
        n257 = event-data() -> ("NewVal"=w388:bool)  [unwired: 1 in]
        n258 = Unbundle("Motor") -> ("Value"=w387:dbl)  [unwired: 1 out]
        n259 = Select(t=w387, s=w388, f=0.0) -> (s? t:f=w385:dbl)
        n260 = call <vilib>:"NT Write Number.vi"("Numeric"=w385, "Name"=w384) -> ()  [unwired: 9 in, 1 out]
      }
      event "Test Slider": Value Change {
        # "When the test mode slider helper is set, update that\ntree row item's value"
        n261 = event-data() -> ("NewVal"=w391:dbl)  [unwired: 1 in]
        n262 = call <vilib>:"NT Write Number.vi"("Numeric"=w391, "Name"=w392) -> ()  [unwired: 9 in, 1 out]
      }
      event "On/Off": Value Change {
        # "When the test mode on/off helper value is set, update that\ntree row item's value"
        n263 = event-data() -> ("NewVal"=w396:bool)  [unwired: 1 in]
        n264 = Boolean To (0,1)(Boolean=w396) -> (0, 1=w395:i16)
        n265 = call <vilib>:"NT Write Number.vi"("Numeric"=w395, "Name"=w394) -> ()  [unwired: 9 in, 1 out]
      }
      event "Rev/Fwd": Value Change {
        # "When the test mode helper value for relays is set, update that\ntree row item's value"
        n266 = event-data() -> ("NewVal.Forward"=w404:bool, "NewVal.Reverse"=w403:bool)  [unwired: 1 in]
        n267 = Boolean To (0,1)(Boolean=w403) -> (0, 1=w402:i16)
        n268 = Boolean To (0,1)(Boolean=w404) -> (0, 1=w400:i16)
        n269 = Negate(x=w402) -> (-x=w401:i16)
        n270 = Add(x=w400, y=w401) -> (x+y=w399:i16)
        n271 = call <vilib>:"NT Write Number.vi"("Numeric"=w399, "Name"=w398) -> ()  [unwired: 9 in, 1 out]
      }
      event "Test Ring": Value Change {
        # "When a test mode helper value is selected from the ring,\nset the tree item's variable to the string value"
        n272 = event-data() -> ("NewVal"=w408:u16)  [unwired: 1 in]
        n273 = property on="Test Ring" class="Ring (strict)"() -> ("Strings []"=w409:string[])  [unwired: 2 in, 2 out]
        n274 = Index Array(array=w409, index=w408) -> (element=w407:string)
        n275 = call <vilib>:"NT Write String.vi"("String"=w407, "Name"=w406) -> ()  [unwired: 9 in, 1 out]
      }
      event "Rec Mode": Value Change {
        # "Update globals for recording mode and path to read log from.\nClear when logging and let NetworkTables set path for vision to\nuse."
        n276 = event-data() -> ("NewVal"=w419:enum32{"Stop", "Record", "Playback"})  [unwired: 1 in]
        n277 = global write "WPI_DashboardLogging Global.vi" "Logging Filename"(path "") -> ()
        n278 = global write "WPI_DashboardLogging Global.vi" "Recording"(w419) -> ()
        n279 = case shown="\"Playback\"" w419 {
          tunnel: w418 -> [_ w421 w429]
          tunnel: [_ _ w428] -> w415
          tunnel: [_ _ w427] -> _
          tunnel: w413 -> [_ _ w425]
          tunnel: cluster{i32, i32} {-250, 170} -> [_ _ w424]
          tunnel: [_ _ T22 {"Image Size"=TRUE, "Image Type"=TRUE, "Pixel Value"=TRUE, "ROI Information"=TRUE, "Zoom Factor"=FALSE} ("Image Information Shown:All Elements")] -> w411
          tunnel: [_ _ TRUE ("Zoom Factor")] -> w410
          frame Default {
          }
          frame "Stop", "Record" {
            # "Place Window too"
            n280 = invoke class="VI" method="FP.Close"(reference=w421) -> (reference out=w420:refnum<vi>)  [unwired: 2 in, 2 out]
            n281 = invoke class="VI" method="Abort VI"(reference=w420) -> ()  [unwired: 2 in, 3 out]
          }
          frame "Playback" {
            n282 = call "Open Playback Panel.vi"("Offset"=w424, "DB VI Ref"=w425, "Playback in"=w429) -> ("Playback out"=w426:refnum<vi>)  [unwired: 8 in]
            n283 = register-events(w426) -> (reference out=w428:refnum<event-registration>, error out=w427:errorcluster)  [unwired: 2 in]
          }
        }
        n284 = property on="Camera Image" class="ImageControl"("Image Information Shown"=w411, "Image Information Visible"=w410) -> ()  [unwired: 2 in, 2 out]
        n285 = call <vilib>:"WPI_DashboardNT Log FieldName Cache.vi"("Operation"=enum16{"Lookup/Add", "Index", "Clear"}."Clear") -> ()  [unwired: 8 in, 3 out]
      }
      event Panel Close {
        w430 = enum32{"Stop", "Record", "Playback"}."Stop" ("Rec Mode")
        # "Playback window has been closed, abort"
        n286 = event-data() -> ()  [unwired: 1 in, 4 out]
        n287 = local write "Rec Mode"(w430) -> ()
        n288 = global write "WPI_DashboardLogging Global.vi" "Recording"(w430) -> ()
      }
      event Panel Close {
        # "Abort playback window and ourself"
        n289 = event-data() -> ()  [unwired: 1 in, 4 out]
        n290 = invoke class="VI" method="FP.Close"(reference=w435) -> (reference out=w434:refnum<vi>)  [unwired: 2 in, 2 out]
        n291 = invoke class="VI" method="Abort VI"(reference=w434) -> (error out=w433:errorcluster)  [unwired: 2 in, 2 out]
        n292 = invoke class="VI" method="Abort VI"(error in=w433) -> ()  [unwired: 2 in, 3 out]
      }
      event "Vision": Value Change {
        # "Enable/Disable Compression slider.\nHW USB is hard-coded into the camera"
        n293 = event-data() -> ("NewVal"=w441:u16)  [unwired: 1 in]
        n294 = Equal?(x=w441, y=u32 2 ("milliseconds to wait")) -> (x = y?=w439:bool)
        n295 = Select(t=T23."Disabled and Grayed Out" ("Disabled"), s=w439, f=T23."Enabled" ("Disabled")) -> (s? t:f=w436:T23)
        n296 = property on="Compression" class="Slide (strict)"("DisabledEnum"=w436) -> ()  [unwired: 2 in, 2 out]
      }
    }
  }
  n297 = while {
    tunnel: w28 -> [w454]
    tunnel: w5 -> [w452]
    tunnel: [w450] -> _
    tunnel: u32 1000 ("milliseconds to wait") -> [w449]
    i -> [w450]
    stop <- FALSE stop-if-true
    n298 = Wait on Notification(notifier=w452, timeout in ms (-1)=w449) -> (notification=w451:string, timed out?=w447:bool)  [unwired: 2 in, 2 out]
    n299 = local read "Rec Mode"() -> (w445:enum32{"Stop", "Record", "Playback"})
    n300 = Equal?(x=w445, y=u16 2 ("Rec Mode")) -> (x = y?=w446:bool)
    n301 = Compound Arithmetic op=OR(invert w447, w446) -> (w448:bool)
    n302 = case shown="True" w448 {
      tunnel: w454 -> [_ w457]
      tunnel: w451 -> [_ w456]
      tunnel: "Dashboard" -> [_ w455]
      frame False {
      }
      frame True {
        n303 = call <vilib>:"Bind Controls to SmartDashboard.vi"("Client Name"=w455, "Bound Control Refs"=w457, "Server IP Address"=w456) -> ()  [unwired: 9 in]
      }
    }
  }
